vi "Read Both Fans Fault and State.vi"(8 "error in (no error)":errorcluster, 11 "HW Dual Fan in":refnum<class "HW Dual Fan.lvclass">) -> (0 "error out":errorcluster, 1 "Fan B Fault":bool, 2 "Fan B State":bool, 3 "Fan A Fault":bool, 5 "Fan A State":bool)   [LabVIEW 2018, in "HW Dual Fan.lvclass"]
uses:
  HW Dual Fan.lvclass
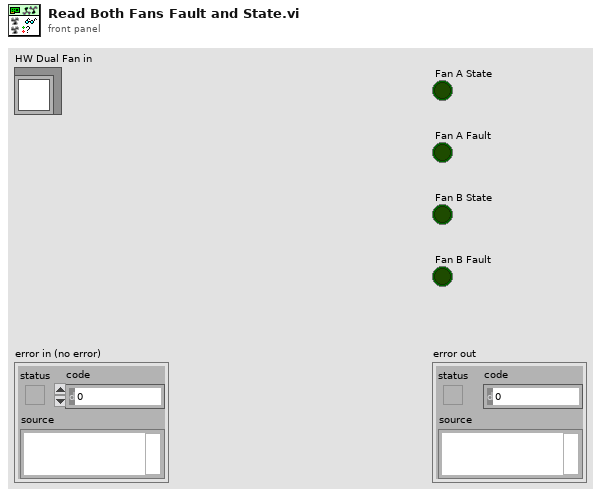
[diagram p1: front panel]
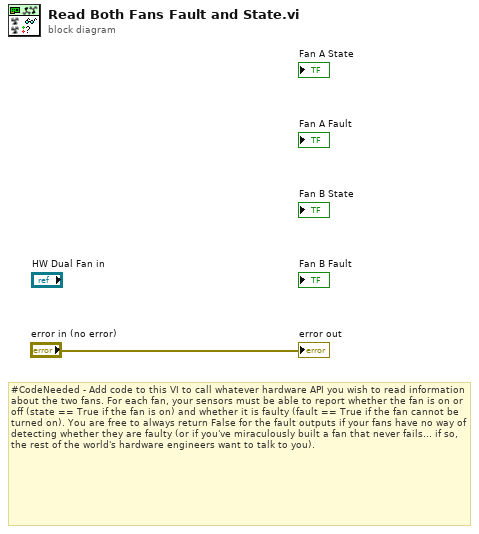
[diagram p0: block diagram]
diagram:
  # "#CodeNeeded - Add code to this VI to call whatever hardware API you wish to read information about the two fans. For each fan, your sensors must be able to report whether the fan is on or off (state == True if the fan is on) and whether it is faulty (fault == True if the fan cannot be turned on). You are free to always return False for the fault outputs if your fans have no way of detecting whether they are faulty (or if you've miraculously built a fan that never fails... if so, the rest of the world's hardware engineers want to talk to you)."
  "error out" <- "error in (no error)"
